vi "EVENT REPORT(SubVI).vi"(10 "all rows":string[](array[string]), 11 "ORDER ID:-":dbl) -> ()   [LabVIEW 2021]
uses:
  <vilib>/Utility/file.llb/Write Delimited Spreadsheet (DBL).vi
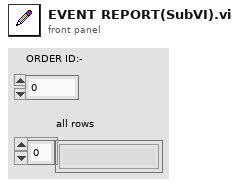
[diagram p1: front panel]
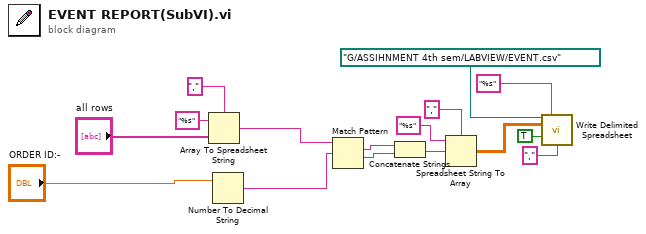
[diagram p0: block diagram]
diagram:
  n1 = Array To Spreadsheet String(delimiter (Tab)=",", array="all rows", 3:"%s" ("format string")) -> (spreadsheet string=w4:string)
  n2 = Number To Decimal String(number="ORDER ID:-") -> (decimal integer string=w6:string)  [unwired: 1 in]
  n3 = Match Pattern(string=w4, regular expression=w6) -> (match substring=w7:string, after substring=w8:string)  [unwired: 1 in, 2 out]
  n4 = Concatenate Strings(w7, w8) -> (w10:string)
  n5 = Spreadsheet String To Array(delimiter (Tab)=",", format string="%s", spreadsheet string=w10) -> (array=w13:dbl[][])  [unwired: 1 in]
  n6 = call-poly <vilib>:"Write Delimited Spreadsheet.vi"("file path (dialog if empty)"=path "G:/ASSIHNMENT 4th sem/LABVIEW/EVENT.csv" ("new file path (Not A Path if cancelled)"), "format (%.3f)"="%s", "2D data"=w13, "append to file? (new file:F)"=TRUE, "delimiter (\\t)"="," ("delimiter (\\t)")) -> ()  [unwired: 9 in, 2 out]
